vi "Close.vi"(8 "error in":errorcluster, 11 "Flow Setpoint in":refnum<class "Flow Setpoint.lvclass">) -> (0 "error out":errorcluster, 3 "Flow Setpoint out":refnum<class "Flow Setpoint.lvclass">)   [LabVIEW 2023, in "Flow Setpoint.lvclass"]
uses:
  Flow Setpoint.lvclass
  Flow Setpoint.lvclass/Flow Setpoint.ctl
  Parents/Setpoint/Setpoint.lvclass
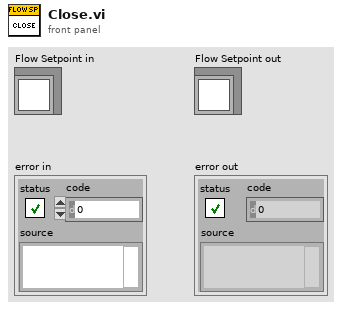
[diagram p1: front panel]
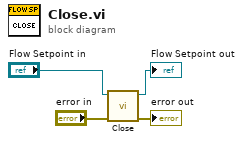
[diagram p0: block diagram]
diagram:
  n1 = call-parent "Close.vi"("error in"="error in", "Setpoint in"="Flow Setpoint in") -> ("error out"=→"error out":errorcluster, "Setpoint out"=→"Flow Setpoint out":refnum<class "Flow Setpoint.lvclass">)  [unwired: 8 in]
